vi "Generate Main Image header file.vi"(8 "error in (no error)":errorcluster, 10 "folders to image header files":path[](array[path])=[path "D:/CASE/Mars Rover/Working Directory/osr-rover-code/OsrScreen/emoji_16x32_source"], 11 "path to main image header file":path=path "D:/CASE/Mars Rover/Working Directory/osr-rover-code/OsrScreen/Osr_Screen_Face.h") -> (0 "error out":errorcluster)   [LabVIEW 2019, in "LabVIEW RGB565 Convertor.lvlib"]
uses:
  LabVIEW RGB565 Convertor.lvlib
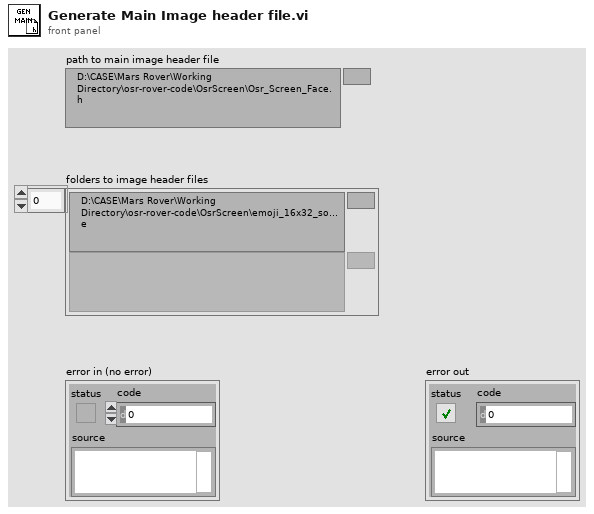
[diagram p1: front panel]
types:
  T1 = enum16{"open", "replace", "create", "open or create", "replace or create", "replace or create with confirmation"}
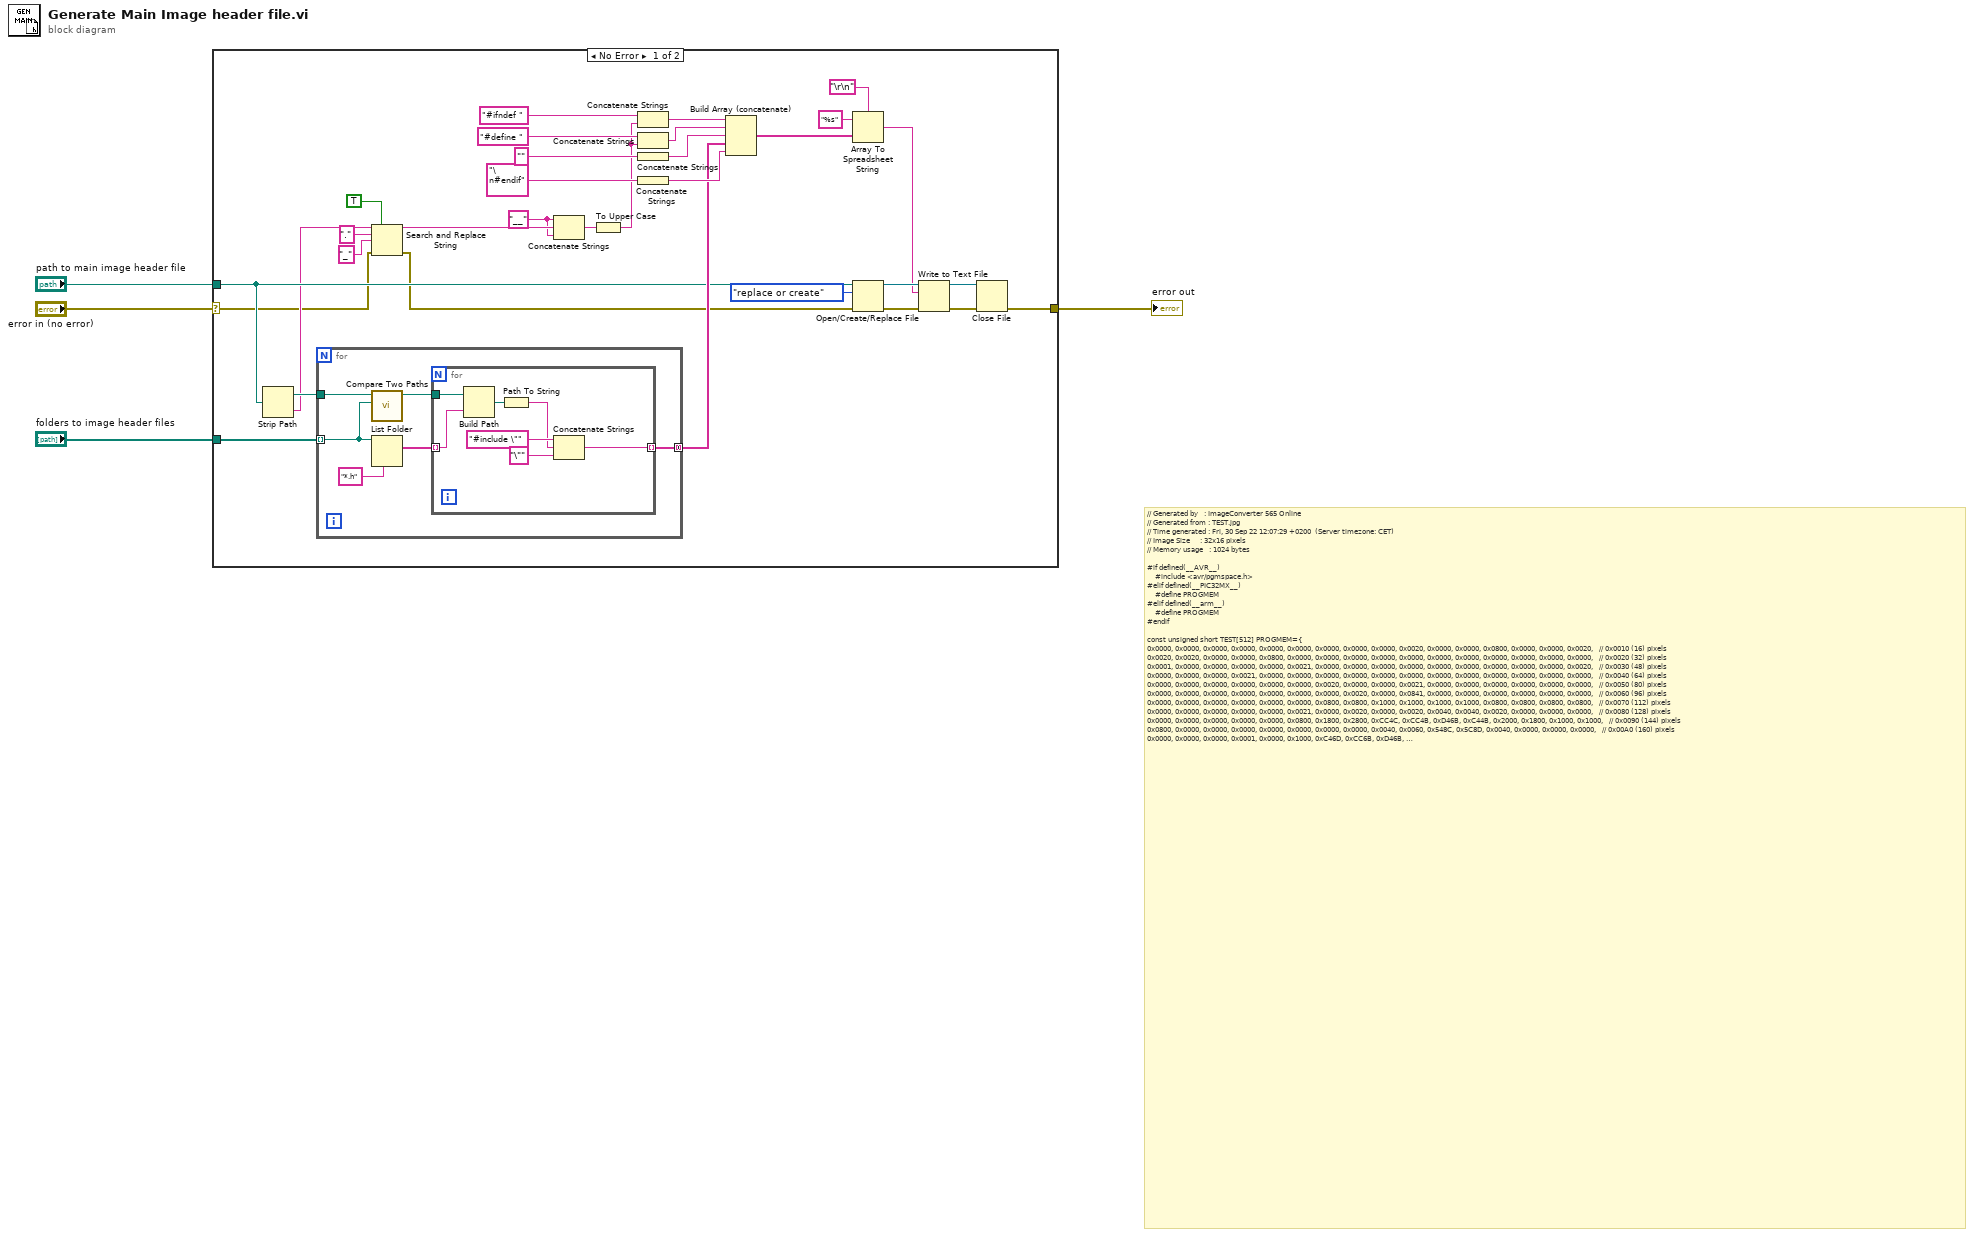
[diagram p0: block diagram]
diagram:
  # "// Generated by   : ImageConverter 565 Online\n// Generated from : TEST.jpg\n// Time generated : Fri, 30 Sep 22 12:07:29 +0200  (Server timezone: CET)\n// Image Size     : 32x16 pixels\n// Memory usage   : 1024 bytes\n\n#if defined(__AVR__)\n    #include <avr/pgmspace.h>\n#elif defined(__PIC32MX__)\n    #define PROGMEM\n#elif defined(__arm__)\n    #define PROGMEM\n#endif\n\nconst unsigned short TEST[512] PROGMEM={\n0x0000, 0x0000, 0x0000, 0x0000, 0x0000, 0x0000, 0x0000, 0x0000, 0x0000, 0x0020, 0x0000, 0x0000, 0x0800, 0x0000, 0x0000, 0x0020,   // 0x0010 (16) pixels\n0x0020, 0x0020, 0x0000, 0x0000, 0x0800, 0x0000, 0x0000, 0x0000, 0x0000, 0x0000, 0x0000, 0x0000, 0x0000, 0x0000, 0x0000, 0x0000,   // 0x0020 (32) pixels\n0x0001, 0x0000, 0x0000, 0x0000, 0x0000, 0x0021, 0x0000, 0x0000, 0x0000, 0x0000, 0x0000, 0x0000, 0x0000, 0x0000, 0x0000, 0x0020,   // 0x0030 (48) pixels\n0x0000, 0x0000, 0x0000, 0x0021, 0x0000, 0x0000, 0x0000, 0x0000, 0x0000, 0x0000, 0x0000, 0x0000, 0x0000, 0x0000, 0x0000, 0x0000,   // 0x0040 (64) pixels\n0x0000, 0x0000, 0x0000, 0x0000, 0x0000, 0x0000, 0x0020, 0x0000, 0x0000, 0x0021, 0x0000, 0x0000, 0x0000, 0x0000, 0x0000, 0x0000,   // 0x0050 (80) pixels\n0x0000, 0x0000, 0x0000, 0x0000, 0x0000, 0x0000, 0x0000, 0x0020, 0x0000, 0x0841, 0x0000, 0x0000, 0x0000, 0x0000, 0x0000, 0x0000,   // 0x0060 (96) pixels\n0x0000, 0x0000, 0x0000, 0x0000, 0x0000, 0x0000, 0x0800, 0x0800, 0x1000, 0x1000, 0x1000, 0x1000, 0x0800, 0x0800, 0x0800, 0x0800,   // 0x0070 (112) pixels\n0x0000, 0x0000, 0x0000, 0x0000, 0x0000, 0x0021, 0x0000, 0x0020, 0x0000, 0x0020, 0x0040, 0x0040, 0x0020, 0x0000, 0x0000, 0x0000,   // 0x0080 (128) pixels\n0x0000, 0x0000, 0x0000, 0x0000, 0x0000, 0x0800, 0x1800, 0x2800, 0xCC4C, 0xCC4B, 0xD46B, 0xC44B, 0x2000, 0x1800, 0x1000, 0x1000,   // 0x0090 (144) pixels\n0x0800, 0x0000, 0x0000, 0x0000, 0x0000, 0x0000, 0x0000, 0x0000, 0x0040, 0x0060, 0x548C, 0x5C8D, 0x0040, 0x0000, 0x0000, 0x0000,   // 0x00A0 (160) pixels\n0x0000, 0x0000, 0x0000, 0x0001, 0x0000, 0x1000, 0xC46D, 0xCC6B, 0xD46B, 0x3000, 0x3800, 0xCC8C, 0xBC8D, 0xB48E, 0xBC8F, 0x1800,   // 0x00B0 (176) pixels\n0x0800, 0x0000, 0x0000, 0x0000, 0x0020, 0x0040, 0x0020, 0x0040, 0x0080, 0x546C, 0x54AD, 0x00A0, 0x0040, 0x0000, 0x0020, 0x0000,   // 0x00C0 (192) pixels\n0x0000, 0x0000, 0x0000, 0x0000, 0x0020, 0x0800, 0xC48D, 0x2800, 0x1800, 0x1000, 0x1000, 0x1000, 0x0800, 0x1000, 0xC48D, 0x2000,   // 0x00D0 (208) pixels\n0x0800, 0x0000, 0x0000, 0x0020, 0x546C, 0x54AD, 0x0060, 0x0060, 0x4C6C, 0x54AD, 0x0060, 0x0020, 0x0000, 0x0000, 0x0000, 0x0000,   // 0x00E0 (224) pixels\n0x0000, 0x0000, 0x0000, 0x0000, 0x0000, 0x0800, 0xBC8D, 0x2000, 0x0800, 0x0000, 0x0000, 0x0800, 0x1000, 0x1800, 0xBC6C, 0x2000,   // 0x00F0 (240) pixels\n0x0800, 0x0000, 0x0000, 0x0040, 0x00E0, 0x44EB, 0x00C0, 0x548D, 0x54AD, 0x00A0, 0x0020, 0x0000, 0x0000, 0x0000, 0x0000, 0x0000,   // 0x0100 (256) pixels\n0x0000, 0x0000, 0x0000, 0x0000, 0x0000, 0x0800, 0xC48D, 0x2000, 0x0000, 0x0020, 0x0000, 0x1000, 0x2800, 0xCC8B, 0xBC6D, 0x1000,   // 0x0110 (272) pixels\n0x0000, 0x0000, 0x0000, 0x0040, 0x00C0, 0x44CB, 0x0100, 0x4CCD, 0x0080, 0x0020, 0x0000, 0x0000, 0x0000, 0x0000, 0x0000, 0x0000,   // 0x0120 (288) pixels\n0x0000, 0x0000, 0x0000, 0x0000, 0x0020, 0x0800, 0xCC6C, 0x2800, 0x0800, 0x0000, 0x0800, 0x2000, 0xCC6B, 0xCC4B, 0x1800, 0x0800,   // 0x0130 (304) pixels\n0x0000, 0x0000, 0x0000, 0x0040, 0x00A0, 0x4CCC, 0x450C, 0x44AC, 0x0040, 0x0000, 0x0000, 0x0000, 0x0000, 0x0000, 0x0000, 0x0000,   // 0x0140 (320) pixels\n0x0000, 0x0000, 0x0000, 0x0000, 0x0000, 0x1000, 0xCC4B, 0x3800, 0x1800, 0xB4AF, 0xBC8D, 0xC46D, 0xC48E, 0x1800, 0x0800, 0x0000,   // 0x0150 (336) pixels\n0x0000, 0x0000, 0x0000, 0x0040, 0x00A0, 0x4CCC, 0x4CEC, 0x00A0, 0x0020, 0x0000, 0x0000, 0x0000, 0x0020, 0x0000, 0x0000, 0x0000,   // 0x0160 (352) pixels\n0x0000, 0x0000, 0x0000, 0x0000, 0x0000, 0x1000, 0xC46D, 0xCC8C, 0x1800, 0x1800, 0x2000, 0x2000, 0x1800, 0x0800, 0x0000, 0x0000,   // 0x0170 (368) pixels\n0x0000, 0x0000, 0x0000, 0x0020, 0x0080, 0x5C8D, 0x544C, 0x0060, 0x0000, 0x0000, 0x0000, 0x0000, 0x0000, 0x0000, 0x0000, 0x0000,   // 0x0180 (384) pixels\n0x0800, 0x0000, 0x0000, 0x0000, 0x0000, 0x0000, 0x0800, 0x1000, 0x0800, 0x0800, 0x1000, 0x0800, 0x0800, 0x0800, 0x0000, 0x0000,   // 0x0190 (400) pixels\n0x0000, 0x0000, 0x0000, 0x0000, 0x0020, 0x0020, 0x0040, 0x0020, 0x0000, 0x0000, 0x0000, 0x0000, 0x0000, 0x0000, 0x0000, 0x0000,   // 0x01A0 (416) pixels\n0x0800, 0x0000, 0x0000, 0x0001, 0x0000, 0x0000, 0x0000, 0x0000, 0x0000, 0x0000, 0x0000, 0x0000, 0x0000, 0x0000, 0x0000, 0x0000,   // 0x01B0 (432) pixels\n0x0020, 0x0000, 0x0000, 0x0000, 0x0000, 0x0000, 0x0000, 0x0000, 0x0000, 0x0000, 0x0000, 0x0000, 0x0000, 0x0000, 0x0000, 0x0000,   // 0x01C0 (448) pixels\n0x0000, 0x0000, 0x0000, 0x0000, 0x0021, 0x0000, 0x0000, 0x0020, 0x0000, 0x0000, 0x0000, 0x0020, 0x0000, 0x0000, 0x0000, 0x0000,   // 0x01D0 (464) pixels\n0x0000, 0x0000, 0x0000, 0x0000, 0x0000, 0x0020, 0x0000, 0x0000, 0x0000, 0x0000, 0x0000, 0x0000, 0x0000, 0x0000, 0x0000, 0x0000,   // 0x01E0 (480) pixels\n0x0000, 0x0000, 0x0000, 0x0020, 0x0000, 0x0020, 0x0000, 0x0000, 0x0000, 0x0000, 0x0020, 0x0000, 0x0000, 0x0000, 0x0000, 0x0000,   // 0x01F0 (496) pixels\n0x0000, 0x0000, 0x0000, 0x0000, 0x0000, 0x0000, 0x0000, 0x0000, 0x0000, 0x0000, 0x0020, 0x0000, 0x0000, 0x0000, 0x0000, 0x0000,   // 0x0200 (512) pixels\n};"
  n1 = case shown="No Error" "error in (no error)" {
    selector: "error in (no error)" -> [w11 w50]
    tunnel: "path to main image header file" -> [w13 _]
    tunnel: "folders to image header files" -> [w32 _]
    tunnel: [w16 w50] -> w2
    frame No Error {
      w5 = "__" ("string")
      n2 = Strip Path(path=w13) -> (stripped path=w14:path, name=w12:string)
      n3 = for {
        tunnel: w32 -> [w38] mode=indexing
        tunnel: [w40] -> w26 mode=concatenating
        tunnel: w14 -> [w37]
        n4 = call <vilib>:"Compare Two Paths.vi"("Path 2"=w38, "Path 1"=w37) -> ("Relative Path from 1 to 2"=w39:path)  [unwired: 6 in, 3 out]
        n5 = List Folder(path=w38, pattern="*.h") -> (filenames=w41:string[])  [unwired: 2 in, 3 out]
        n6 = for {
          tunnel: w41 -> [w45] mode=indexing
          tunnel: [w47] -> w40 mode=indexing
          tunnel: w39 -> [w46]
          n7 = Build Path(base path=w46, name or relative path=w45) -> (appended path=w44:path)
          n8 = Path To String(path=w44) -> (string=w43:string)
          n9 = Concatenate Strings("#include \"" ("string"), w43, "\"" ("string")) -> (w47:string)
        }
      }
      n10 = Search and Replace String(replace all?=TRUE ("replace all? (F)"), input string=w12, search string=".", replace string="_" ("replace string (\"\")"), error in=w11) -> (result string=w6:string, error out=w10:errorcluster)  [unwired: 3 in, 2 out]
      n11 = Concatenate Strings(w5, w6, w5) -> (w34:string)
      n12 = To Upper Case(1:w34) -> (0:w15:string)
      n13 = Concatenate Strings("#ifndef " ("string"), w15) -> (w31:string)
      n14 = Concatenate Strings("#define " ("string"), w15) -> (w29:string)
      n15 = Concatenate Strings("" ("string")) -> (w28:string)
      n16 = Concatenate Strings("\n#endif" ("string")) -> (w27:string)
      n17 = Build Array (concatenate)(w31, w29, w28, w26, w27) -> (w23:string[])
      n18 = Array To Spreadsheet String(delimiter (Tab)="\r\n", array=w23, 3:"%s" ("format string")) -> (spreadsheet string=w17:string)
      n19 = Open/Create/Replace File(file path (use dialog)=w13, error in=w10, operation (0:open)=T1."replace or create") -> (refnum out=w20:refnum<file>, error out=w19:errorcluster)  [unwired: 3 in, 1 out]
      n20 = Write to Text File(file (use dialog)=w20, text=w17, error in=w19) -> (refnum out=w21:refnum<file>, error out=w22:errorcluster)  [unwired: 1 in, 1 out]
      n21 = Close File(refnum=w21, error in=w22) -> (error out=w16:errorcluster)  [unwired: 1 out]
    }
    frame Error {
    }
  }
  "error out" <- w2
